vi "MultiScale Wavelet LL SubVI.vi"(8 "error in (no error)":errorcluster, 10 "Image Dst":T1, 11 "Image Src":T1) -> (0 "error out":errorcluster, 3 "Image Dst Out":T1)   [LabVIEW 2023]
uses:
  WaveLet Param Cluster Typedef.ctl
  <vilib>/vision/Image Controls.llb/IMAQ Image.ctl
  db40c56f-7327-4ec9-8689-6ae8bd04cb59.vi
  <vilib>/addons/_Advanced Signal Processing/NI_AdvSigProcWA.lvlib
panel:
  in  "Overall Contrast":dbl=0.7
  in  "Multiplier":dbl[](array[slide])=[220.55384826660156, 212.6769256591797, 192.984619140625, 252.06153869628906, 283.5692443847656, 319.015380859375, 252.06153869628906, 236.3076934814453, 181.1692352294922, 110.27692413330078, 129.96923076923076, 102.4000015258789] scale=0.0..512.0
  in  "Power":dbl[](array[slide])=[0.38461539149284363, 0.4307692348957062, 0.38461539149284363, 0.5230769515037537, 0.42307692766189575, 0.5538461804389954, 0.6461538672447205, 0.6153846383094788, 0.6153846383094788, 0.6000000238418579, 0.4000000059604645, 0.4000000059604645] scale=0.0..2.0
  out "Levels":i32=9
  in  "Multipliers":T2[][](array[typedef])=[[{"Multiplier"=0.5}, {"Multiplier"=0.45}, {"Multiplier"=0.5}], [{"Multiplier"=1.0}, {"Multiplier"=1.0}, {"Multiplier"=1.0}], [{"Multiplier"=1.0}, {"Multiplier"=1.0}, {"Multiplier"=1.0}], [{"Multiplier"=1.0}, {"Multiplier"=1.0}, {"Multiplier"=1.0}], [{"Multiplier"=1.0}, {"Multiplier"=1.0}, {"Multiplier"=1.0}], [{"Multiplier"=1.0}, {"Multiplier"=1.0}, {"Multiplier"=1.0}], [{"Multiplier"=1.0}, {"Multiplier"=1.0}, {"Multiplier"=1.0}], [{"Multiplier"=1.0}, {"Multiplier"=1.0}, {"Multiplier"=1.0}], [{"Multiplier"=1.0}, {"Multiplier"=1.0}, {"Multiplier"=1.0}], [{"Multiplier"=1.0}, {"Multiplier"=1.0}, {"Multiplier"=1.0}]]
  in  "Wavelet":u16(ring) items=["db02"=0, "db03"=1, "db04"=2, "db05"=3, "db06"=4, "db07"=5, "db08"=6, "db09"=7, "db10"=8, "db11"=9, "db12"=10, "db13"=11, "db14"=12, "Haar"=13, "bior1_3"=14, "bior1_5"=15, "bior2_2"=16, "bior2_4"=17, "bior2_6"=18, "bior2_8"=19, "bior3_1"=20, "bior3_3"=21, "bior3_5"=22, "bior3_7"=23, "bior3_9"=24, "bior4_4 (FBI)"=25, "bior5_5"=38, "bior6_8"=39, "coif1"=26, "coif2"=27, "coif3"=28, "coif4"=29, "coif5"=30, "sym2"=31, "sym3"=32, "sym4"=33, "sym5"=34, "sym6"=35, "sym7"=36, "sym8"=37]
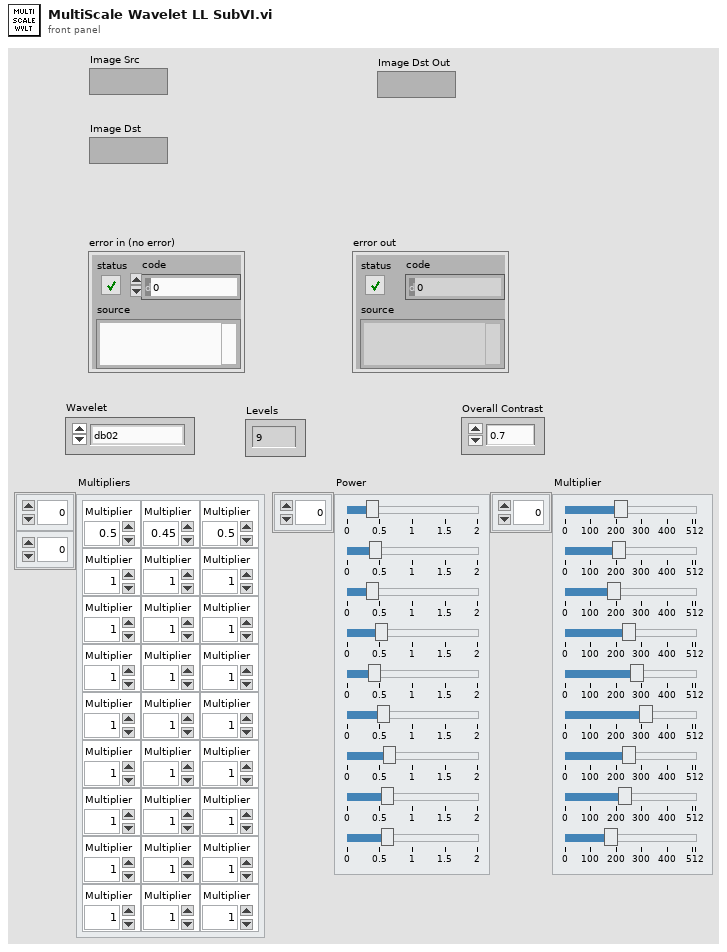
[diagram p1: front panel]
types:
  T1 = typedef "IMAQ Image.ctl" = refnum<image>
  T2 = typedef "WaveLet Param Cluster Typedef.ctl" = cluster{"Multiplier":dbl}
  T3 = cluster{"low_low":dbl[][], "low_high":dbl[][], "high_low":dbl[][], "high_high":dbl[][]}[]
  T4 = cluster{"low_low":dbl[][], "low_high":dbl[][], "high_low":dbl[][], "high_high":dbl[][]}
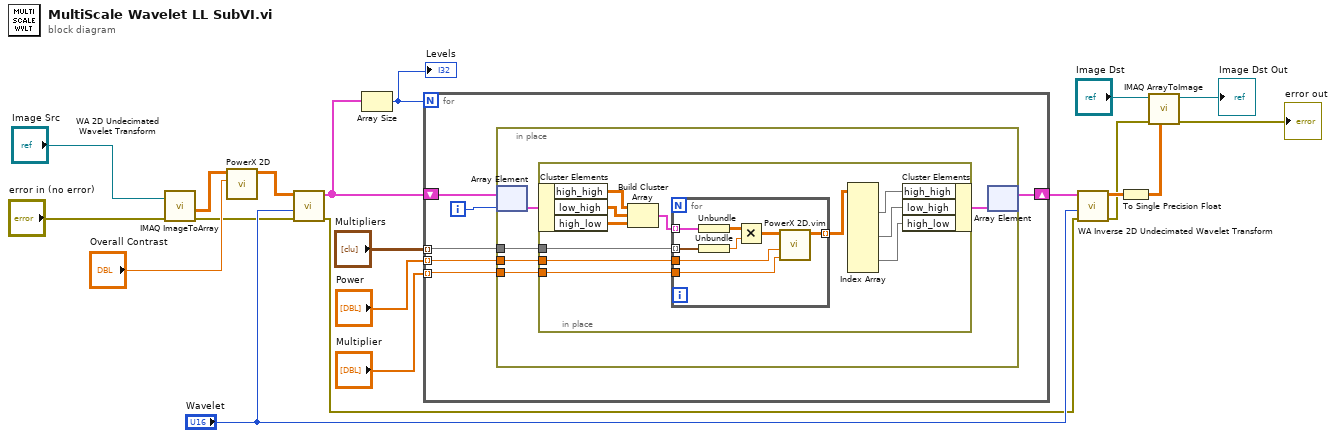
[diagram p0: block diagram]
diagram:
  n1 = call "IMAQ ImageToArray"("error in (no error)"="error in (no error)", "Image"="Image Src") -> ("Image Pixels (Float)"=w18:sgl[][], "error out"=w3:errorcluster)  [unwired: 2 in, 3 out]
  n2 = call "PowerX 2D.vi"("Power"="Overall Contrast", "Signal In"=w18) -> ("Signal Out"=w15:dbl[][])  [unwired: 9 in]
  n3 = call <vilib>:"WA 2D Undecimated Wavelet Transform.vi"("error in (no error)"=w3, "wavelet"="Wavelet", "signal"=w15) -> ("error out"=w2:errorcluster, "UWT coef"=w10:T3)  [unwired: 2 in, 5 out]
  n4 = Array Size(array=w10) -> (size(s)=w6:i32)
  "Levels" <- w6
  n5 = for {
    N: w6 -> [_]
    shift-right: [w21] -> w9
    shift-left: w10 -> [w23]
    tunnel: "Multipliers" -> [w26] mode=indexing
    tunnel: "Power" -> [w25] mode=indexing
    tunnel: "Multiplier" -> [w24] mode=indexing
    i -> [w22]
    n6 = in-place {
      in-place-border: w26 -> [w31]
      in-place-border: w25 -> [w30]
      in-place-border: w24 -> [w29]
      n7 = in-place-array #1(w23, w22) -> (w28:T4)
      n8 = in-place {
        in-place-border: w31 -> [w40]
        in-place-border: w30 -> [w39]
        in-place-border: w29 -> [w38]
        n9 = in-place-cluster #2(w28) -> ("high_high"=w37:dbl[][], "low_high"=w36:dbl[][], "high_low"=w35:dbl[][])
        n10 = Build Cluster Array(w37, w36, w35) -> (w42:cluster{"high_low":dbl[][]}[])
        n11 = for {
          tunnel: w42 -> [w50] mode=indexing
          tunnel: [w44] -> w41 mode=indexing
          tunnel: w40 -> [w48] mode=indexing
          tunnel: w39 -> [w43]
          tunnel: w38 -> [w45]
          n12 = Unbundle(w50) -> ("high_low"=w49:dbl[][])
          n13 = Unbundle(w48) -> ("Multiplier"=w47:dbl)
          n14 = Multiply(x=w49, y=w47) -> (x*y=w46:dbl[][])
          n15 = call "PowerX 2D.vim"("Multiplier"=w45, "Power"=w43, "Signal In"=w46) -> ("Signal Out"=w44:dbl[][])  [unwired: 8 in]
        }
        n16 = Index Array(array=w41) -> (element #1=w34:dbl[][], element #2=w33:dbl[][], element #3=w32:dbl[][])  [unwired: 9 in]
        n17 = in-place-cluster #2("high_high"=w34, "low_high"=w33, "high_low"=w32) -> (w27:T4)
      }
      n18 = in-place-array #1(w27) -> (w21:T3)  [unwired: 1 out]
    }
  }
  n19 = call <vilib>:"WA Inverse 2D Undecimated Wavelet Transform.vi"("error in (no error)"=w2, "wavelet"="Wavelet", "UWT coef"=w9) -> ("error out"=w1:errorcluster, "signal"=w7:dbl[][])  [unwired: 1 in, 6 out]
  n20 = To Single Precision Float(number=w7) -> (single precision float=w16:sgl[][])
  n21 = call "IMAQ ArrayToImage"("Image Pixels (Float)"=w16, "error in (no error)"=w1, "Image"="Image Dst") -> ("error out"=→"error out":errorcluster, "Image Out"=→"Image Dst Out":T1)  [unwired: 7 in]
